vi "Execute Program.vi"(4 "error in (no error)":errorcluster, 6 "Program Name":string, 7 "VISA resource name":refnum<visa-resource-name>) -> (0 "error out":errorcluster, 3 "VISA resource name out":refnum<visa-resource-name>)   [LabVIEW 2018, in "Newport ESP301.lvlib"]
doc: "This command is used to start executing a program. When the command is\nreceived the controller executes the program line by line or according to the flow control instructions.\nDuring program execution, only commands that ask for information and that stop the motion are still allowed. Any of the following commands will terminate a program, in one way or another: AB, AP, MF, RS and ST. Most natural way to just stop a program execution is by using the AP command, the other ones having a more drastic effect."
uses:
  Newport ESP301.lvlib
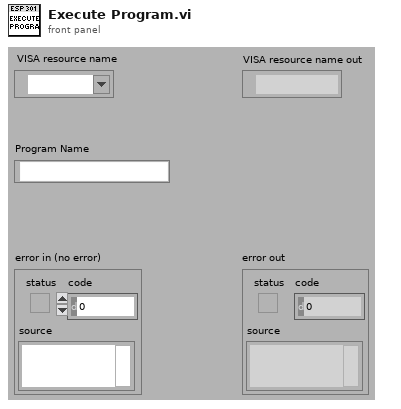
[diagram p1: front panel]
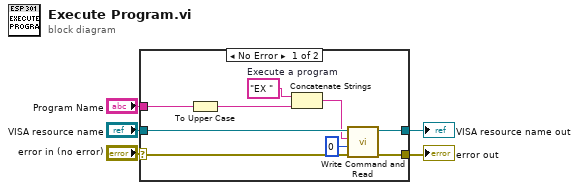
[diagram p0: block diagram]
diagram:
  n1 = case shown="No Error" "error in (no error)" {
    selector: "error in (no error)" -> [w11 w16]
    tunnel: [w13 w16] -> w5
    tunnel: "VISA resource name" -> [w14 w15]
    tunnel: [w12 w15] -> w4
    tunnel: "Program Name" -> [w7 _]
    frame No Error {
      w8 = "EX "  # Execute a program
      n2 = To Upper Case(1:w7) -> (0:w6:string)
      n3 = Concatenate Strings(w8, w6) -> (w10:string)
      n4 = call "Write Command and Read.vi"("error in (no error)"=w11, "Bytes to read (100)"=u32 0, "Command"=w10, "VISA resource name"=w14) -> ("error out"=w13:errorcluster, "VISA resource name out"=w12:refnum<visa-resource-name>)  [unwired: 3 in, 1 out]
    }
    frame Error {
    }
  }
  "error out" <- w5
  "VISA resource name out" <- w4
